vi "I2C_HostWriteCMD-ParamMemory_2.vi"(8 "error in":errorcluster, 10 "CMD-Param_Bytes":u8[](array[numeric]), 11 "FPGA VI Reference In":T1) -> (0 "error out":errorcluster, 3 "FPGA VI Reference Out":T1)   [LabVIEW 2019]
doc: "Updates the 'Write' memory block on the FPGA with the Command bytes. The update is done a byte at a time. When the update is complete the Execute boolean is set on the FPGA to execute the command. \n\nVI Written By:\nPeter Fuller\nSenior Engineer\nplf Consulting, LLC"
uses:
  <vilib>/rvi/interface/nirviReadWriteControl/nirviReadWriteControl.xnode
  Controls/FPGA_Reference.ctl
  FPGA Bitfiles/LS_Durability_FPGA_9627.lvbitx
  <vilib>/rvi/errors/niLvFpgaMergeErrorWithErrorCode.vi
  <vilib>/rvi/errors/niLvFpgaAdjustHostInterfaceError.vi
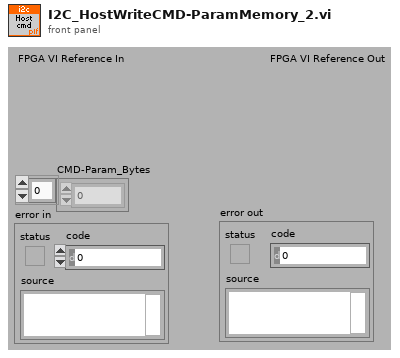
[diagram p1: front panel]
types:
  T1 = typedef "FPGA_Reference.ctl" = refnum<k20>
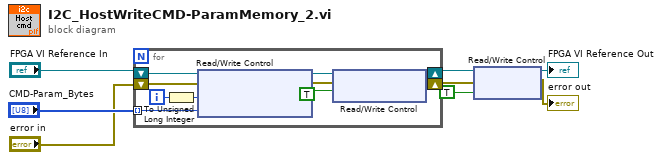
[diagram p0: block diagram]
diagram:
  n1 = for {
    shift-right: [w11] -> w6
    shift-left: "FPGA VI Reference In" -> [w18]
    shift-right: [w9] -> w7
    shift-left: "error in" -> [w17]
    tunnel: "CMD-Param_Bytes" -> [w14] mode=indexing
    i -> [w16]
    n2 = To Unsigned Long Integer(number=w16) -> (unsigned 32bit integer=w15:u32)
    n3 = xnode "Read/Write Control"("FPGA VI Reference In"=w18, "error in"=w17, "MemoryAddress 2"=w15, "CMD/Param 2"=w14) -> ("FPGA VI Reference Out"=w12:T1, "error out"=w10:errorcluster)
    n4 = xnode "Read/Write Control"("FPGA VI Reference In"=w12, "error in"=w10, "UpdateWrite 2"=TRUE ("UpdateWrite")) -> ("FPGA VI Reference Out"=w11:T1, "error out"=w9:errorcluster)
  }
  n5 = xnode "Read/Write Control"("FPGA VI Reference In"=w6, "error in"=w7, "Execute 2"=TRUE ("Execute")) -> ("FPGA VI Reference Out"=→"FPGA VI Reference Out":T1, "error out"=→"error out":errorcluster)
